vi "IV_curve_measurement2.vi"() -> ()   [LabVIEW 2015]
panel:
  in  "Delta":refnum<visa-resource-name>="GPIB0::20::INSTR"
  out "concatenated string":string
  out "error out":errorcluster
  in  "milliseconds to wait":u32=500
  out "IV Curve":cluster{dbl[], dbl[]}(graph)
  in  "IV converter":refnum<visa-resource-name>="GPIB0::20::INSTR"
  in  "Lock in":refnum<visa-resource-name>="GPIB0::5::INSTR"
  out "Actual Voltage":dbl
  in  "Voltage Step (V)":dbl=0.1
  in  "Max Voltage (V)":dbl=1.0
  in  "Min Voltage (V)":dbl
  in  "stop":bool
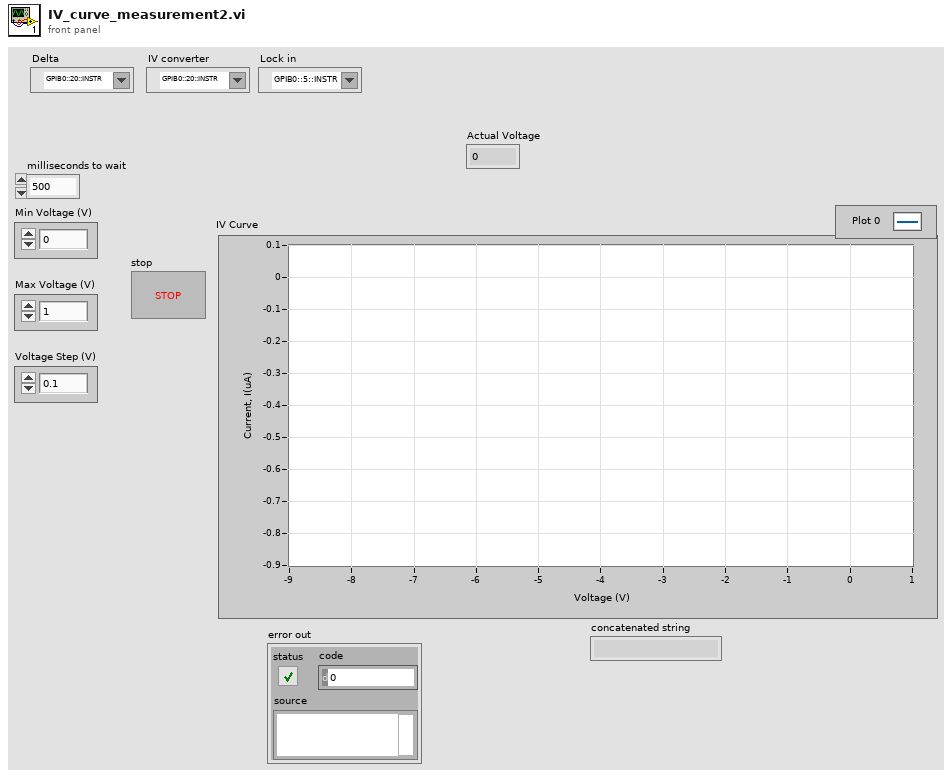
[diagram p1: front panel]
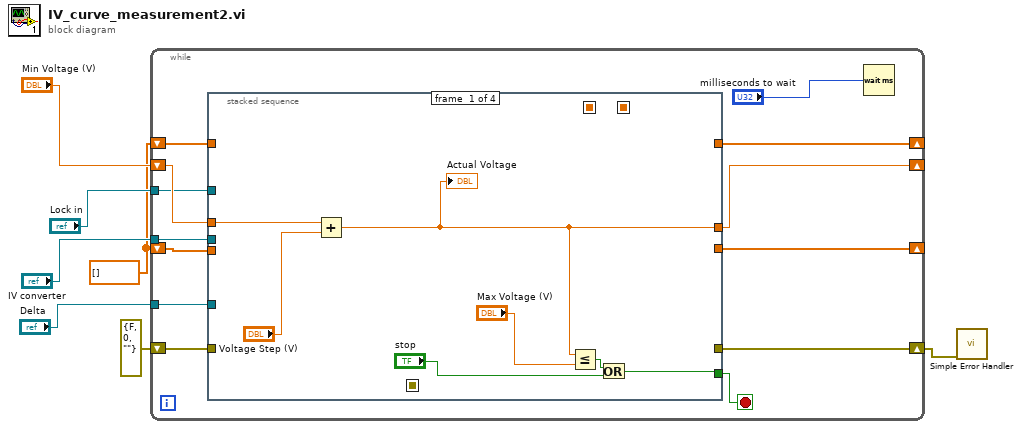
[diagram p0: block diagram]
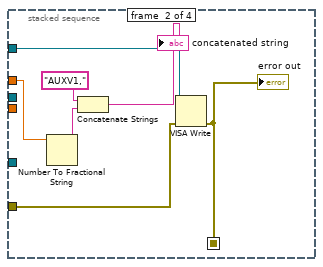
[diagram p2: hidden frame]
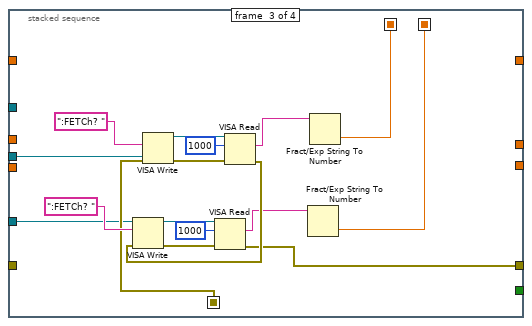
[diagram p3: hidden frame]
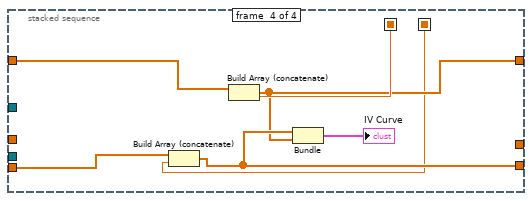
[diagram p4: hidden frame]
diagram:
  w3 = dbl[] []
  n1 = while {
    shift-right: [w18] -> _
    shift-left: "Min Voltage (V)" -> [w19]
    tunnel: "Lock in" -> [w17]
    shift-right: [w14] -> w2
    shift-left: errorcluster {"status"=FALSE, "code"=0, "source"=""} ("error out") -> [w16]
    tunnel: "IV converter" -> [w15]
    shift-right: [w13] -> _
    shift-left: w3 -> [w12]
    shift-right: [w11] -> _
    shift-left: w3 -> [w10]
    tunnel: "Delta" -> [w8]
    stop <- w20 stop-if-true
    n2 = stacked-sequence {
      seq-local: [_ w28 _ _] -> [_ _ w38 _]
      seq-local: [_ _ w45 _] -> [_ _ _ w57]
      seq-local: [_ _ w35 _] -> [_ _ _ w52]
      tunnel: [w26 _ _ _] -> w20
      tunnel: w19 -> [w25 w34 _ _]
      tunnel: [w23 _ _ _] -> w18
      tunnel: w17 -> [_ w33 _ _]
      tunnel: w16 -> [_ w29 _ _]
      tunnel: w15 -> [_ _ w49 _]
      tunnel: [_ _ w39 _] -> w14
      tunnel: [_ _ _ w55] -> w13
      tunnel: w12 -> [_ _ _ w58]
      tunnel: [_ _ _ w54] -> w11
      tunnel: w10 -> [_ _ _ w56]
      tunnel: w8 -> [_ _ w37 _]
      frame #0 {
        n3 = Add(x=w25, y="Voltage Step (V)") -> (x+y=w23:dbl)
        "Actual Voltage" <- w23
        n4 = Less Or Equal?(x=w23, y="Max Voltage (V)") -> (x <= y?=w27:bool)
        n5 = Or(x=w27, y="stop") -> (x .or. y?=w26:bool)
      }
      frame #1 {
        n6 = Number To Fractional String(number=w34) -> (F-format string=w31:string)  [unwired: 3 in]
        n7 = Concatenate Strings("AUXV1," ("string"), w31) -> (w30:string)
        "concatenated string" <- w30
        n8 = VISA Write(VISA resource name=w33, write buffer=w30, error in (no error)=w29) -> (error out=w28:errorcluster)  [unwired: 2 out]
        "error out" <- w28
      }
      frame #2 {
        n9 = VISA Write(VISA resource name=w49, write buffer=":FETCh? " ("data"), error in (no error)=w38) -> (VISA resource name out=w48:refnum<visa-resource-name>, error out=w50:errorcluster)  [unwired: 1 out]
        n10 = VISA Read(VISA resource name=w48, byte count=u32 1000, error in (no error)=w50) -> (read buffer=w46:string, error out=w40:errorcluster)  [unwired: 2 out]
        n11 = VISA Write(VISA resource name=w37, write buffer=":FETCh? " ("data"), error in (no error)=w40) -> (VISA resource name out=w43:refnum<visa-resource-name>, error out=w42:errorcluster)  [unwired: 1 out]
        n12 = VISA Read(VISA resource name=w43, byte count=u32 1000, error in (no error)=w42) -> (read buffer=w36:string, error out=w39:errorcluster)  [unwired: 2 out]
        n13 = Fract/Exp String To Number(string=w36) -> (number=w35:dbl)  [unwired: 3 in, 1 out]
        n14 = Fract/Exp String To Number(string=w46) -> (number=w45:dbl)  [unwired: 3 in, 1 out]
      }
      frame #3 {
        n15 = Build Array (concatenate)(w58, w52) -> (w55:dbl[])
        n16 = Build Array (concatenate)(w56, w57) -> (w54:dbl[])
        n17 = Bundle(w55, w54) -> (→"IV Curve":cluster{dbl[], dbl[]})  [unwired: 1 in]
      }
    }
    n18 = Wait (ms)(milliseconds to wait="milliseconds to wait") -> ()  [unwired: 1 out]
  }
  n19 = call <vilib>:"Simple Error Handler.vi"("error in (no error)"=w2) -> ()  [unwired: 4 in, 5 out]
